vi "gfitsio-get-names-cols.vi"(8 "error in (no error)":errorcluster, 11 "gfits refnum":T1) -> (0 "error out":errorcluster, 1 "number of columns":i32, 2 "column names":string[](array[string]), 3 "dup gfits refnum":T1)   [LabVIEW 2023, in "gfitsio.lvlib"]
doc: "Get the number of columns in the current FITS table."
uses:
  gfitsio.lvlib
  gfitsio-refnum.ctl
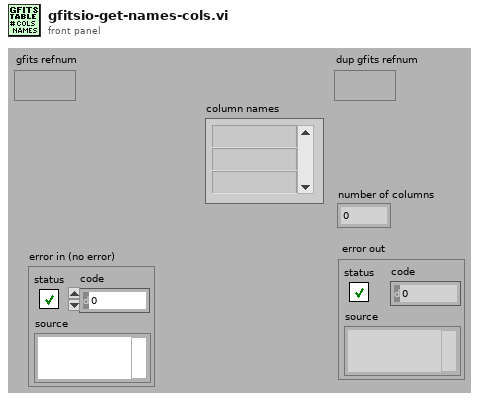
[diagram p1: front panel]
types:
  T1 = typedef "gfitsio.lvlib/gfitsio-refnum.ctl" = refnum<k1>
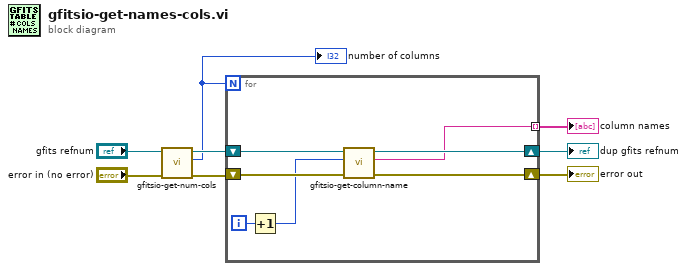
[diagram p0: block diagram]
diagram:
  n1 = call "gfitsio-get-num-cols.vi"("error in (no error)"="error in (no error)", "gfits refnum"="gfits refnum") -> ("error out"=w5:errorcluster, "number of columns"=w1:i32, "dup gfits refnum"=w6:T1)  [unwired: 7 in]
  "number of columns" <- w1
  n2 = for {
    N: w1 -> [_]
    shift-right: [w11] -> w3
    shift-left: w6 -> [w15]
    shift-right: [w10] -> w2
    shift-left: w5 -> [w14]
    tunnel: [w9] -> w4 mode=indexing
    i -> [w13]
    n3 = Increment(x=w13) -> (x+1=w12:i32)
    n4 = call "gfitsio-get-column-name.vi"("error in (no error)"=w14, "column number"=w12, "Refnum in"=w15) -> ("error out"=w10:errorcluster, "column name"=w9:string, "Refnum out"=w11:T1)  [unwired: 6 in]
  }
  "error out" <- w2
  "dup gfits refnum" <- w3
  "column names" <- w4
